vi "Walsh Hadamard.vi"(0 "X":dbl[](array[numeric])) -> (1 "Walsh Hadamard {X}":dbl[](array[numeric]), 2 "error":i32)   [LabVIEW 2014, in "NI_Gmath.lvlib"]
doc: "Computes the real Walsh Hadamard transform of the input sequence <B>X</B>."
uses:
  NI_Gmath.lvlib
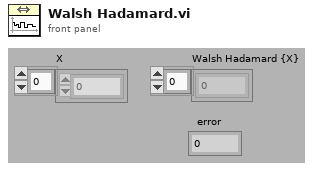
[diagram p1: front panel]
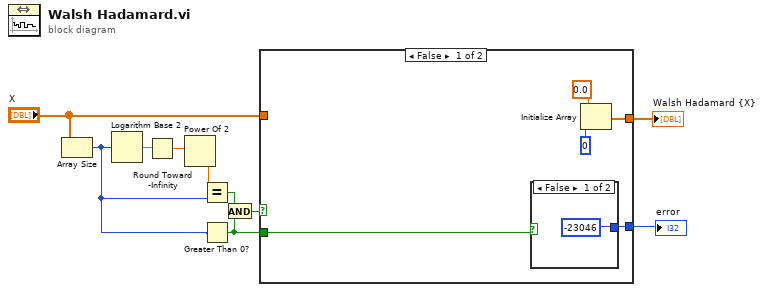
[diagram p0: block diagram]
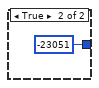
[diagram p2: hidden frame]
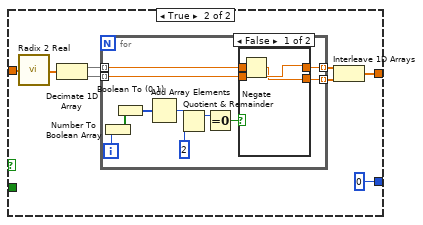
[diagram p3: hidden frame]
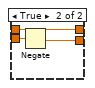
[diagram p4: hidden frame]
diagram:
  n1 = Array Size(array="X") -> (size(s)=w2:i32)
  n2 = Logarithm Base 2(1:w2) -> (0:w7:dbl)
  n3 = Round Toward -Infinity(1:w7) -> (0:w6:dbl)
  n4 = Power Of 2(x=w6) -> (2^x=w5:dbl)
  n5 = Equal?(x=w5, y=w2) -> (x = y?=w4:bool)
  n6 = Greater Than 0?(x=w2) -> (x > 0?=w1:bool)
  n7 = And(x=w4, y=w1) -> (x .and. y?=w3:bool)
  n8 = case shown="False" w3 {
    tunnel: "X" -> [_ w25]
    tunnel: [w13 w19] -> w9
    tunnel: [w12 0] -> w8
    tunnel: w1 -> [w11 _]
    frame False {
      n9 = case shown="False" w11 {
        tunnel: [-23046 -23051] -> w12
        frame False {
        }
        frame True {
        }
      }
      n10 = Initialize Array(0.0, 0) -> (w13:dbl[])
    }
    frame True {
      n11 = call "Radix 2 Real.vi"("X"=w25) -> ("Y"=w20:dbl[])
      n12 = Decimate 1D Array(w20) -> (w21:dbl[], w22:dbl[])
      n13 = for {
        tunnel: w21 -> [w29] mode=indexing
        tunnel: w22 -> [w28] mode=indexing
        tunnel: [w27] -> w23 mode=indexing
        tunnel: [w26] -> w24 mode=indexing
        i -> [w36]
        n14 = Number To Boolean Array(number=w36) -> (Boolean array=w35:bool[])
        n15 = Boolean To (0,1)(Boolean=w35) -> (0, 1=w34:i16[])
        n16 = Add Array Elements(numeric array=w34) -> (sum=w32:i16)
        n17 = Quotient & Remainder(x=w32, y=2) -> (x-y*floor(x/y)=w31:i32)  [unwired: 1 out]
        n18 = Equal To 0?(x=w31) -> (x = 0?=w30:bool)
        n19 = case shown="False" w30 {
          tunnel: w29 -> [w39 w42]
          tunnel: w28 -> [w38 w41]
          tunnel: [w38 w42] -> w27
          tunnel: [w37 w40] -> w26
          frame False {
            n20 = Negate(x=w39) -> (-x=w37:dbl)
          }
          frame True {
            n21 = Negate(x=w41) -> (-x=w40:dbl)
          }
        }
      }
      n22 = Interleave 1D Arrays(w23, w24) -> (w19:dbl[])
    }
  }
  "Walsh Hadamard {X}" <- w9
  "error" <- w8
